vi "compress to 8 bit slow.vi"(8 "error in (no error)":errorcluster, 9 "Image Dst Out":T1, 10 "Custom Data Out":string, 11 "Refnum in":T1) -> (0 "error out":errorcluster, 1 "Numeric 2":dbl, 2 "Numeric":u32, 3 "Refnum out":T1)   [LabVIEW 2020]
uses:
  <vilib>/vision/Image Controls.llb/IMAQ Image.ctl
  <resource>/objmgr/IMAQImage.rc
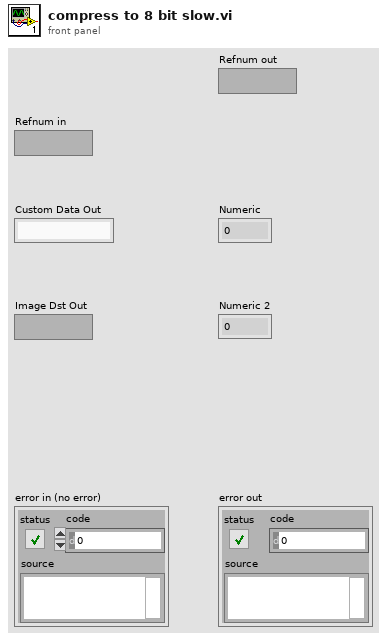
[diagram p1: front panel]
types:
  T1 = typedef "IMAQ Image.ctl" = refnum<image>
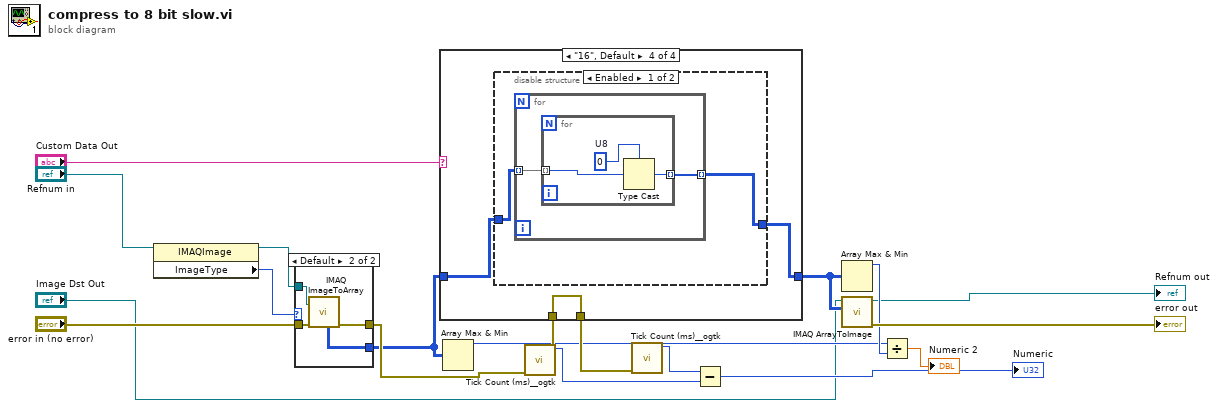
[diagram p0: block diagram]
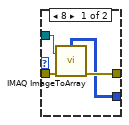
[diagram p2: hidden frame]
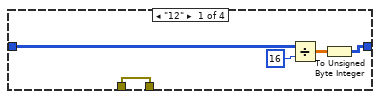
[diagram p3: hidden frame]
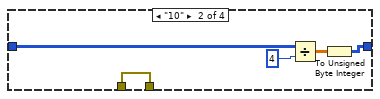
[diagram p4: hidden frame]
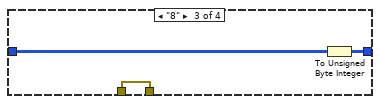
[diagram p5: hidden frame]
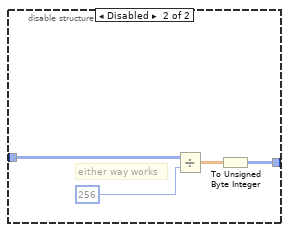
[diagram p6: hidden frame]
diagram:
  n1 = property class="IMAQImage"(reference="Refnum in") -> (reference out=w11:T1, "ImageType"=w12:u32)  [unwired: 1 in, 1 out]
  n2 = case shown="Default" w12 {
    tunnel: [w23 w27] -> w14
    tunnel: "error in (no error)" -> [w22 w26]
    tunnel: [w20 w25] -> w4
    tunnel: w11 -> [w21 w24]
    frame 8 {
      n3 = call "IMAQ ImageToArray"("error in (no error)"=w22, "Image"=w21) -> ("error out"=w23:errorcluster, "Image Pixels (U8)"=w20:u8[][])  [unwired: 2 in, 3 out]
    }
    frame Default {
      n4 = call "IMAQ ImageToArray"("error in (no error)"=w26, "Image"=w24) -> ("Image Pixels (U16)"=w25:u16[][], "error out"=w27:errorcluster)  [unwired: 2 in, 3 out]
    }
  }
  n5 = Array Max & Min(array=w4) -> (max value=w6:u16)  [unwired: 3 out]
  n6 = call <userlib>:"Tick Count (ms)__ogtk.vi"("error in (no error)"=w14) -> ("error out"=w15:errorcluster, "millisecond timer value"=w18:u32)  [unwired: 9 in]
  n7 = case shown="\"16\", Default" "Custom Data Out" {
    tunnel: [w29 w34 w40 w43] -> w5
    tunnel: w4 -> [w32 w37 w39 w42]
    tunnel: w15 -> [w28 w33 w38 w41]
    tunnel: [w28 w33 w38 w41] -> w19
    frame "12" {
      n8 = Divide(x=w32, y=16) -> (x/y=w30:dbl[][])
      n9 = To Unsigned Byte Integer(number=w30) -> (unsigned 8bit integer=w29:u8[][])
    }
    frame "10" {
      n10 = Divide(x=w37, y=4) -> (x/y=w35:dbl[][])
      n11 = To Unsigned Byte Integer(number=w35) -> (unsigned 8bit integer=w34:u8[][])
    }
    frame "8" {
      n12 = To Unsigned Byte Integer(number=w39) -> (unsigned 8bit integer=w40:u8[][])
    }
    frame "16", Default {
      n13 = disable-structure shown="Enabled" {
        disable-tunnel: [w45 w51] -> w43
        disable-tunnel: w42 -> [w44 w52]
        frame Enabled {
          n14 = for {
            tunnel: w44 -> [w47] mode=indexing
            tunnel: [w46] -> w45 mode=indexing
            n15 = for {
              tunnel: w47 -> [w49] mode=indexing
              tunnel: [w48] -> w46 mode=indexing
              w50 = u8 0  # U8
              n16 = Type Cast(type=w50, x=w49) -> (*(type *) &x=w48:u8)
            }
          }
        }
        frame Disabled {
          # "either way works"
          n17 = Divide(x=w52, y=256) -> (x/y=w53:dbl[][])
          n18 = To Unsigned Byte Integer(number=w53) -> (unsigned 8bit integer=w51:u8[][])
        }
      }
    }
  }
  n19 = call <userlib>:"Tick Count (ms)__ogtk.vi"("error in (no error)"=w19) -> ("millisecond timer value"=w17:u32)  [unwired: 9 in, 1 out]
  n20 = Subtract(x=w17, y=w18) -> (x-y=→"Numeric":u32)
  n21 = Array Max & Min(array=w5) -> (max value=w7:u8)  [unwired: 3 out]
  n22 = call "IMAQ ArrayToImage"("Image Pixels (U8)"=w5, "Image"="Image Dst Out") -> ("error out"=→"error out":errorcluster, "Image Out"=→"Refnum out":T1)  [unwired: 8 in]
  n23 = Divide(x=w6, y=w7) -> (x/y=→"Numeric 2":dbl)
